vi "Request Event.vi"(0 "connection info":T1, 5 "State Variables":T3, 7 "Address Lookup Table":variant, 9 "PGN":u32, 11 "DA":u8(ring), 12 "Error Q":refnum<queue>, 13 "VI Ref":refnum<vi>) -> (4 "connection info":T1, 6 "Response":string, 8 "Address Lookup Table Out":variant)   [LabVIEW 2015, in "J1939 Addon Shared.lvlib"]
uses:
  J1939 Addon Shared.lvlib
  Types/Private Data.ctl
  Types/Error Cluster.ctl
  Types/Error Types.ctl
  <vilib>/NI/STM/TCP/TCP Connection Info.ctl
  <vilib>/NI/STM/SubVIs/MetaDataElement.ctl
  <vilib>/NI/STM/NI STM.lvlib
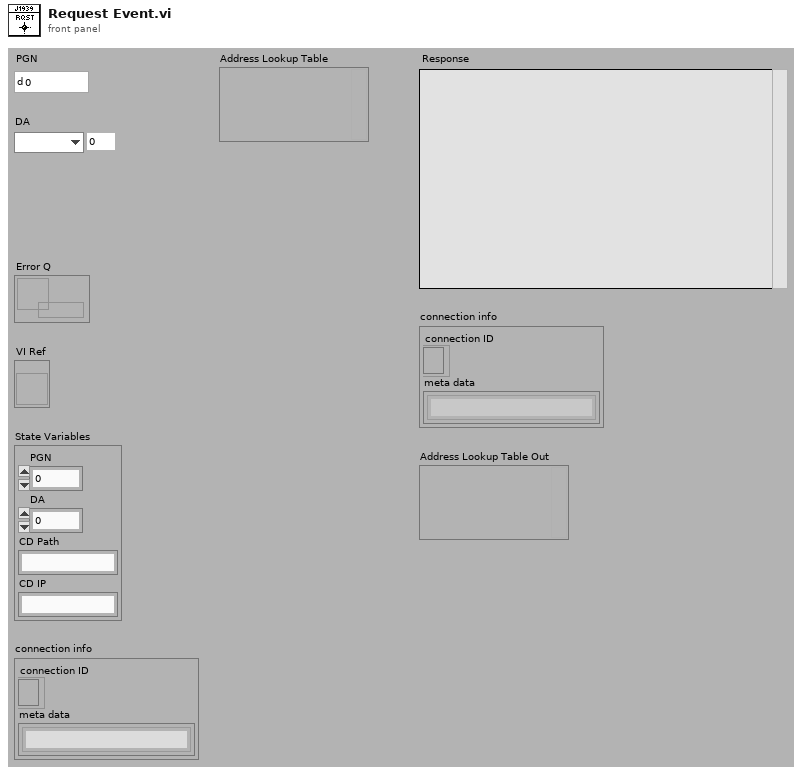
[diagram p1: front panel]
types:
  T1 = typedef "NI STM.lvlib/TCP Connection Info.ctl" = cluster{"connection ID":refnum<k5>, "meta data":T2[]}
  T2 = typedef "NI STM.lvlib/MetaDataElement.ctl" = string
  T3 = typedef "J1939 Addon Shared.lvlib/Private Data.ctl" = cluster{"PGN":u32, "DA":u8, "CD Path":string, "CD IP":string}
  T4 = typedef "J1939 Addon Shared.lvlib/Error Types.ctl" = enum16{"Request", "RAW Generation", "Clear Active DTCs", "Clear Previous DTCs", "Addresses", "TLAs", "Get Active DTCs", "Get Previous DTCs", "TCP Connection"}
  T5 = typedef "XNET Frame CAN.ctl" = cluster{"timestamp":timestamp, "payload":u8[], "identifier":u32, "type":T6, "extended?":bool, "echo?":bool}
  T6 = typedef "XNET Frame Type CAN.ctl" = u8
  T7 = typedef "J1939 Addon Shared.lvlib/Error Cluster.ctl" = cluster{"error out":errorcluster, "Enum":T4, "Address":u8, "Timestamp":timestamp}
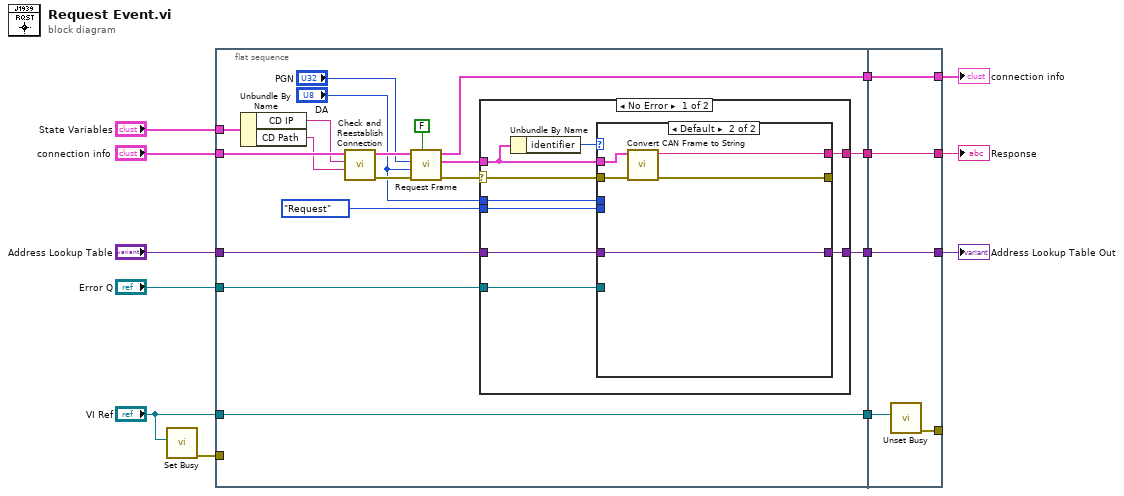
[diagram p0: block diagram]
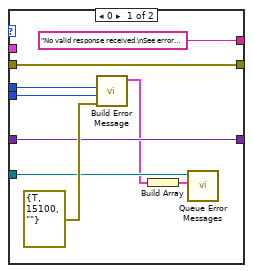
[diagram p2: hidden frame]
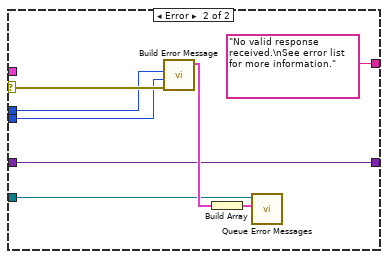
[diagram p3: hidden frame]
diagram:
  n1 = call <vilib>:"Set Busy.vi"("VI reference (current VI)"="VI Ref") -> ("error out"=w4:errorcluster)  [unwired: 9 in, 1 out]
  n2 = flat-sequence {
    tunnel: "connection info" -> [w27]
    tunnel: w4 -> [_]
    tunnel: [w23] -> w13
    tunnel: "Error Q" -> [w25]
    tunnel: "Address Lookup Table" -> [w21]
    tunnel: [w22] -> w12
    tunnel: [w20] -> w11
    tunnel: "State Variables" -> [w17]
    tunnel: [w14] -> w10
    tunnel: "VI Ref" -> [w14]
    tunnel: [w67] -> w3
    tunnel: w13 -> [w67]
    tunnel: [w66] -> _
    tunnel: w12 -> [w65]
    tunnel: [w65] -> w7
    tunnel: w11 -> [w63]
    tunnel: w10 -> [w64]
    tunnel: [w63] -> w1
    frame #0 {
      n3 = Unbundle By Name(w17) -> ("CD IP"=w16:string, "CD Path"=w15:string)
      n4 = call "Check and Reestablish Connection.vi"("CD Path"=w15, "IP Address"=w16, "connection info"=w27) -> ("error out"=w31:errorcluster, "connection info"=w30:T1)  [unwired: 7 in]
      n5 = call "Request Frame.vi"("Ignore Response"=FALSE, "error in (no error)"=w31, "DA"="DA", "PGN"="PGN", "connection info"=w30) -> ("error out"=w29:errorcluster, "Response Frame"=w28:T5, "connection info"=w23:T1)  [unwired: 4 in]
      n6 = case shown="No Error" w29 {
        selector: w29 -> [w40 w59]
        tunnel: w28 -> [w38 _]
        tunnel: [w39 "No valid response received.\nSee error list for more information." ("String")] -> w20
        tunnel: w25 -> [w33 w60]
        tunnel: Error_Types."Request" ("Enum") -> [w36 w58]
        tunnel: [w35 w57] -> w22
        tunnel: w21 -> [w34 w57]
        tunnel: "DA" -> [w32 w56]
        frame No Error {
          n7 = Unbundle By Name(w38) -> ("identifier"=w37:u32)
          n8 = case shown="Default" w37 {
            tunnel: [w49 w54] -> _
            tunnel: w38 -> [_ w53]
            tunnel: w40 -> [w49 w52]
            tunnel: ["No valid response received.\nSee error list for more information." ("String") w51] -> w39
            tunnel: w32 -> [w47 _]
            tunnel: w36 -> [w46 _]
            tunnel: [w45 w50] -> w35
            tunnel: w34 -> [w45 w50]
            tunnel: w33 -> [w43 _]
            frame 0 {
              n9 = call "Build Error Message.vi"("error IO"=errorcluster {"status"=TRUE, "code"=15100, "source"=""}, "Enum"=w46, "Address"=w47) -> ("Error Cluster"=w42:T7)  [unwired: 8 in]
              n10 = Build Array(w42) -> (w44:T7[])
              n11 = call "Queue Error Messages.vi"("Error Array"=w44, "queue out"=w43) -> ()  [unwired: 9 in, 1 out]
            }
            frame Default {
              n12 = call "Convert CAN Frame to String.vi"("error in"=w52, "element"=w53) -> ("error out"=w54:errorcluster, "String"=w51:string)  [unwired: 8 in]
            }
          }
        }
        frame Error {
          n13 = call "Build Error Message.vi"("error IO"=w59, "Enum"=w58, "Address"=w56) -> ("Error Cluster"=w62:T7)  [unwired: 8 in]
          n14 = Build Array(w62) -> (w61:T7[])
          n15 = call "Queue Error Messages.vi"("Error Array"=w61, "queue out"=w60) -> ()  [unwired: 9 in, 1 out]
        }
      }
    }
    frame #1 {
      n16 = call <vilib>:"Unset Busy.vi"("VI reference (current VI)"=w64) -> ("error out"=w66:errorcluster)  [unwired: 10 in]
    }
  }
  "Address Lookup Table Out" <- w7
  "connection info" <- w3
  "Response" <- w1
